vi "plc ios.vi"(7 "Calibpath":path=path "D:/Data Break Padel Test Rig/config/Calib/Calib_Date.txt", 8 "error In":errorcluster, 11 "connection ID IN":refnum<k5>) -> (0 "error out":errorcluster, 3 "connection ID OUT":refnum<k5>)   [LabVIEW 2015]
uses:
  Calibration/calibration.ctl
panel:
  out "PLC INPUT":T1
  out "PLC OUTPUT":T2
  out "Data":u32[](array[numeric])
  in  "Stop Button":bool
  # "PLC I/O's Detail"
  # "X40\tSATRT PB\nX41\tEMERGENYY PB\nX42\tRESET PB\nX43\tHOME PB\nX44\tCONTROL ON SIGNAL\nX45\tAIR PRESSURE SIGNAL\nX46\tSAFETY SENSOR SIGNAL-1\nX47\tSAFETY SENSOR SIGNAL-2\nX48\tPART PRESENMT SENSOR\nX49\tCLAMP CYL-1 UP RS\nX4A\tCLAMP CYL-1 DWN RS\nX4B\tCLAMP CYL-2 UP RS\nX4C\tCLAMP CYL-2 DWN RS\nX4D\tSPRING HOLD CYL FWD RS\nX4E\tSPRING HOLD CYL REV RS\nX4F\tSLIDE CYL UP RS\nX50\tSLIDE CYL DWN RS\nX51\tFRONT SIMULATOR REV RS\nX52\tBACK SIMULATOR REV RS\nX53\tSERVO HOMING SENSOR\nX54\tSERVO FWD OVER TRAVEL\nX55\tSERVO REV OVER TRAVEL\nX56\tSERVO FAULT SIGNAL\nX57\tPANEL DOOR OPEN SIGNAL\nX58\tSPARE\nX59\tSPARE\nX5A\tSPARE\nX5B\tSPARE\nX5C\tSPARE\nX5D\tSPARE\nX5E\tSPARE\nX5F\tSPARE"
  # "ATMA AUTOTECH ENGINEERS PVT. LTD."
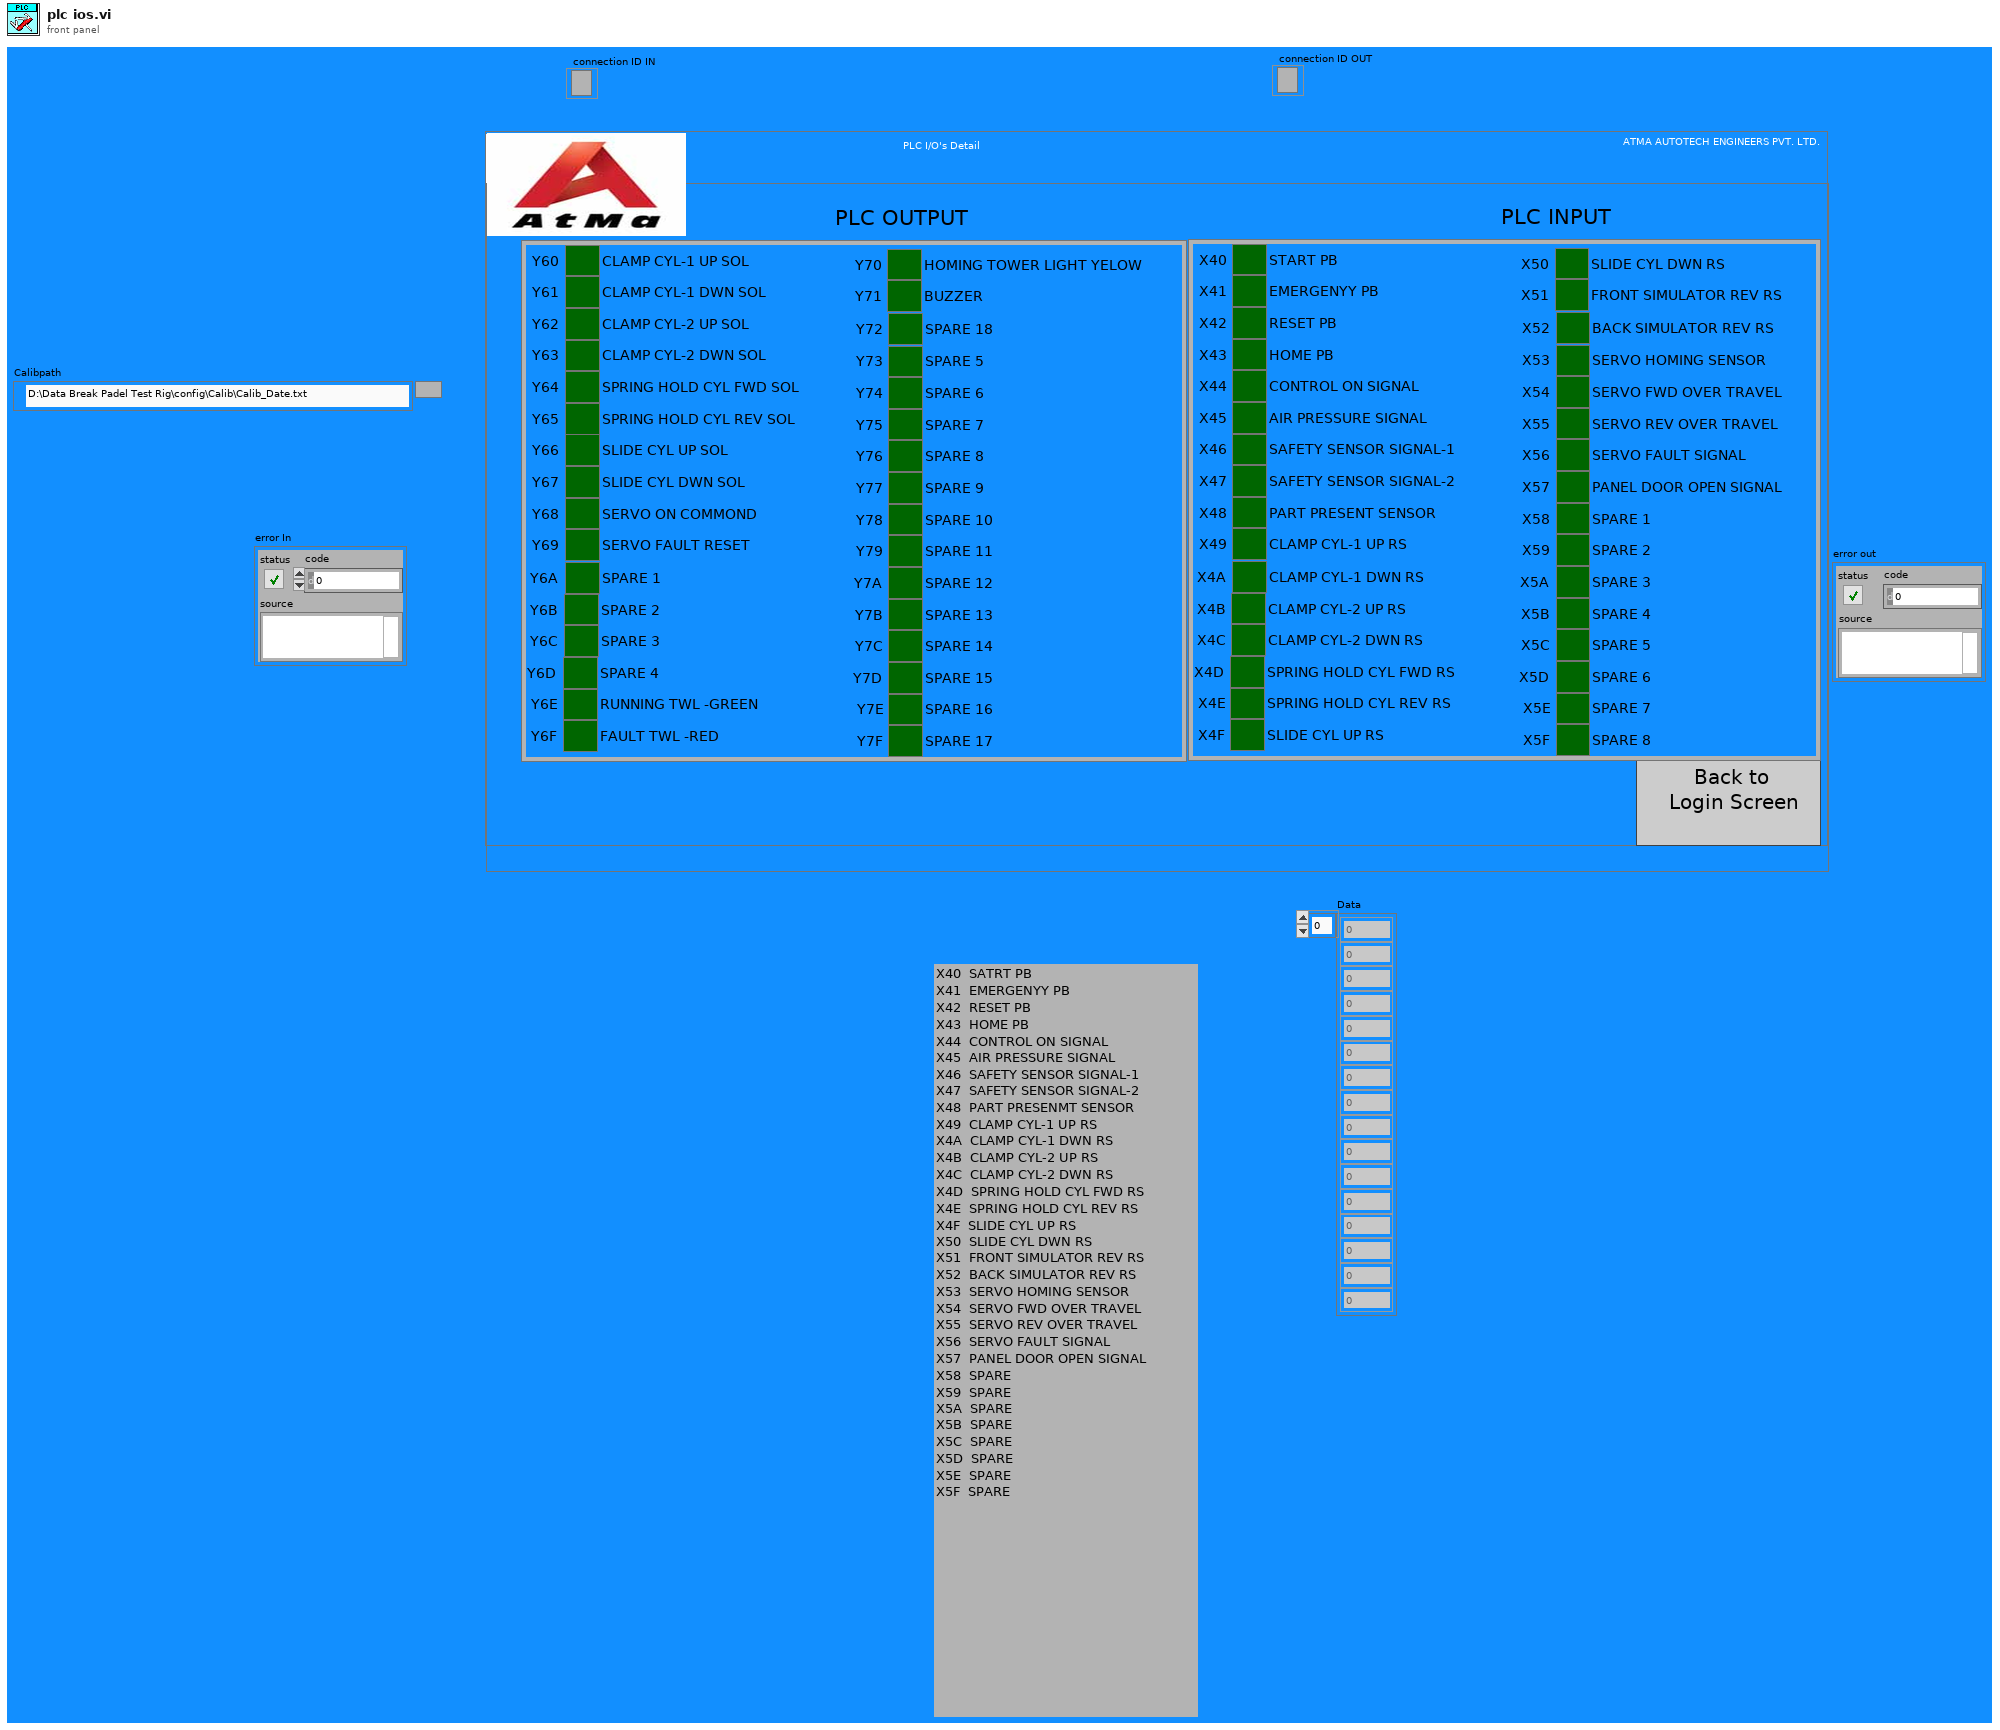
[diagram p1: front panel]
types:
  T1 = cluster{"START PB":bool, "EMERGENYY PB":bool, "RESET PB":bool, "HOME PB":bool, "CONTROL ON SIGNAL":bool, "AIR PRESSURE SIGNAL":bool, "SAFETY SENSOR SIGNAL-1":bool, "SAFETY SENSOR SIGNAL-2":bool, "PART PRESENT SENSOR":bool, "CLAMP CYL-1 UP RS":bool, "CLAMP CYL-1 DWN RS":bool, "CLAMP CYL-2 UP RS":bool, "CLAMP CYL-2 DWN RS":bool, "SPRING HOLD CYL FWD RS":bool, "SPRING HOLD CYL REV RS":bool, "SLIDE CYL UP RS":bool, "SLIDE CYL DWN RS":bool, "FRONT SIMULATOR REV RS":bool, "BACK SIMULATOR REV RS":bool, "SERVO HOMING SENSOR":bool, "SERVO FWD OVER TRAVEL":bool, "SERVO REV OVER TRAVEL":bool, "SERVO FAULT SIGNAL":bool, "PANEL DOOR OPEN SIGNAL":bool, "SPARE 1":bool, "SPARE 2":bool, "SPARE 3":bool, "SPARE 4":bool, "SPARE 5":bool, "SPARE 6":bool, "SPARE 7":bool, "SPARE 8":bool}
  T2 = cluster{"CLAMP CYL-1 UP SOL":bool, "CLAMP CYL-1 DWN SOL":bool, "CLAMP CYL-2 UP SOL":bool, "CLAMP CYL-2 DWN SOL":bool, "SPRING HOLD CYL FWD SOL":bool, "SPRING HOLD CYL REV SOL":bool, "SLIDE CYL UP SOL":bool, "SLIDE CYL DWN SOL":bool, "SERVO ON COMMOND":bool, "SERVO FAULT RESET":bool, "SPARE 1":bool, "SPARE 2":bool, "SPARE 3":bool, "SPARE 4":bool, "RUNNING TWL -GREEN":bool, "FAULT TWL -RED":bool, "HOMING TOWER LIGHT YELOW ":bool, "BUZZER":bool, "SPARE 18":bool, "SPARE 5":bool, "SPARE 6":bool, "SPARE 7":bool, "SPARE 8":bool, "SPARE 9":bool, "SPARE 10":bool, "SPARE 11":bool, "SPARE 12":bool, "SPARE 13":bool, "SPARE 14":bool, "SPARE 15":bool, "SPARE 16":bool, "SPARE 17":bool}
  T3 = typedef "calibration.ctl" = cluster{"Pressing Load":cluster{"Rating":dbl, "Multiplier":dbl, "Offset":dbl}, "Front Break Load":cluster{"Rating":dbl, "Multiplier":dbl, "Offset":dbl}, "Rear Break Load":cluster{"Rating":dbl, "Multiplier":dbl, "Offset":dbl}, "Front Break LVDT":cluster{"Rating":dbl, "Multiplier":dbl, "Offset":dbl}, "Rear Break LVDT":cluster{"Rating":dbl, "Multiplier":dbl, "Offset":dbl}, "AI 5":cluster{"Rating":dbl, "Multiplier":dbl, "Offset":dbl}, "AI 6":cluster{"Rating":dbl, "Multiplier":dbl, "Offset":dbl}, "AI 7":cluster{"Rating":dbl, "Multiplier":dbl, "Offset":dbl}}
  T4 = enum16{"open", "replace", "create", "open or create", "replace or create", "replace or create with confirmation"}
  T5 = cluster{"Rating":dbl, "Multiplier":dbl, "Offset":dbl}
  T6 = cluster{"DI 0-31[0]":bool, "DI 0-31[1]":bool, "DI 0-31[2]":bool, "DI 0-31[3]":bool, "DI 0-31[4]":bool, "DI 0-31[5]":bool, "DI 0-31[6]":bool, "DI 0-31[7]":bool, "DI 0-31[8]":bool, "DI 0-31[9]":bool, "DI 0-31[10]":bool, "DI 0-31[11]":bool, "DI 0-31[12]":bool, "DI 0-31[13]":bool, "DI 0-31[14]":bool, "DI 0-31[15]":bool, "DI 0-31[16]":bool, "DI 0-31[17]":bool, "DI 0-31[18]":bool, "DI 0-31[19]":bool, "DI 0-31[20]":bool, "DI 0-31[21]":bool, "DI 0-31[22]":bool, "DI 0-31[23]":bool, "DI 0-31[24]":bool, "DI 0-31[25]":bool, "DI 0-31[26]":bool, "DI 0-31[27]":bool, "DI 0-31[28]":bool, "DI 0-31[29]":bool, "DI 0-31[30]":bool, "DI 0-31[31]":bool}
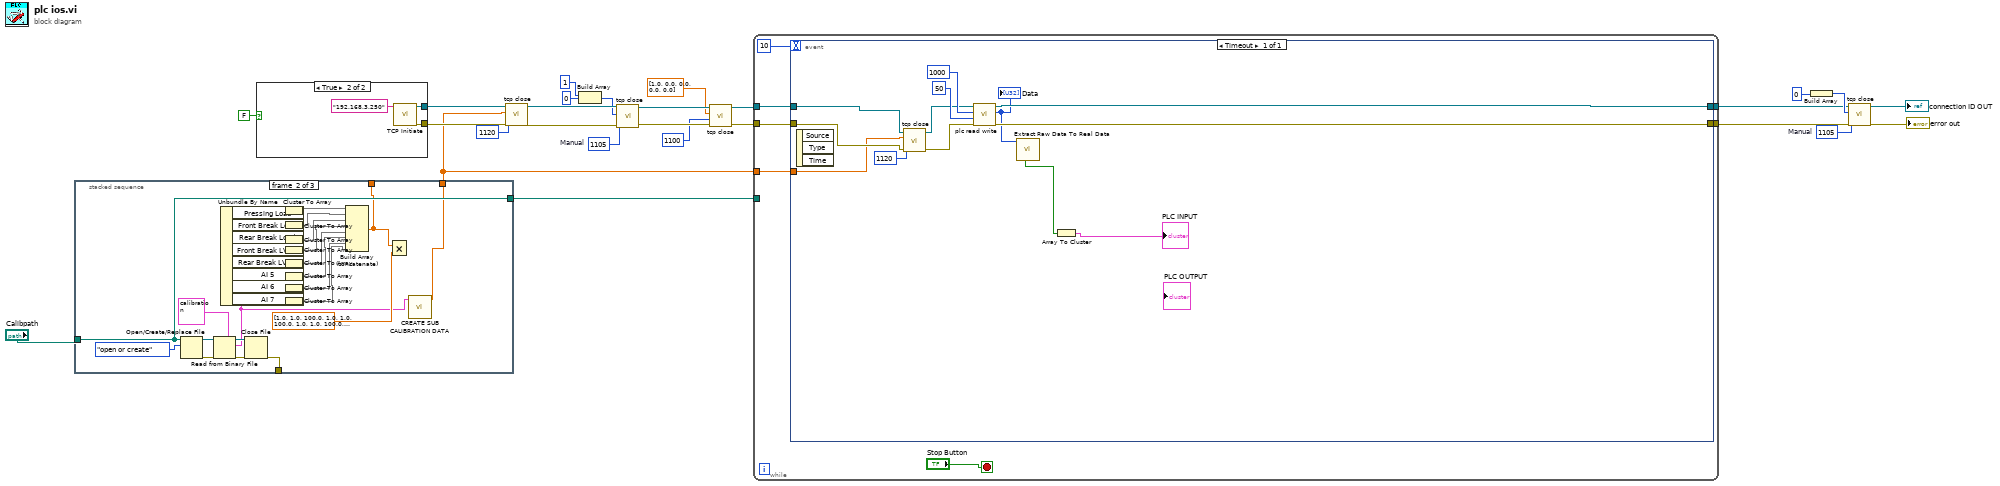
[diagram p0: block diagram]
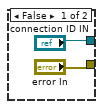
[diagram p2: hidden frame]
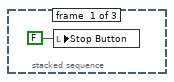
[diagram p3: hidden frame]
diagram:
  w11 = 1105  # Manual
  w19 = 1105  # Manual
  n1 = stacked-sequence {
    tunnel: "Calibpath" -> [_ w48 _]
    tunnel: [_ w48 _] -> w24
    tunnel: [_ w47 _] -> _
    tunnel: [_ w30 _] -> _
    tunnel: [_ w27 _] -> w6
    frame #0 {
      n2 = local write "Stop Button"(FALSE ("Stop Button")) -> ()
    }
    frame #1 {
      n3 = Open/Create/Replace File(file path (use dialog)=w48, operation (0:open)=T4."open or create") -> (refnum out=w52:refnum<file>, error out=w50:errorcluster)  [unwired: 4 in, 1 out]
      n4 = Read from Binary File(5:T3 {"Pressing Load"={"Rating"=0.0, "Multiplier"=0.0, "Offset"=0.0}, "Front Break Load"={"Rating"=0.0, "Multiplier"=0.0, "Offset"=0.0}, "Rear Break Load"={"Rating"=0.0, "Multiplier"=0.0, "Offset"=0.0}, "Front Break LVDT"={"Rating"=0.0, "Multiplier"=0.0, "Offset"=0.0}, "Rear Break LVDT"={"Rating"=0.0, "Multiplier"=0.0, "Offset"=0.0}, "AI 5"={"Rating"=0.0, "Multiplier"=0.0, "Offset"=0.0}, "AI 6"={"Rating"=0.0, "Multiplier"=0.0, "Offset"=0.0}, "AI 7"={"Rating"=0.0, "Multiplier"=0.0, "Offset"=0.0}} ("output cluster"), 8:w50, 11:w52) -> (0:w51:errorcluster, 2:w28:T3, 3:w53:refnum<file>)  [unwired: 3 in, 1 out]
      n5 = Unbundle By Name(w28) -> ("Pressing Load"=w46:T5, "Front Break Load"=w45:T5, "Rear Break Load"=w44:T5, "Front Break LVDT"=w43:T5, "Rear Break LVDT"=w39:T5, "AI 5"=w40:T5, "AI 6"=w41:T5, "AI 7"=w42:T5)
      n6 = Close File(refnum=w53, error in=w51) -> (error out=w47:errorcluster)  [unwired: 1 out]
      n7 = Cluster To Array(cluster=w46) -> (array=w38:dbl[])
      n8 = Cluster To Array(cluster=w45) -> (array=w37:dbl[])
      n9 = Cluster To Array(cluster=w44) -> (array=w36:dbl[])
      n10 = Cluster To Array(cluster=w43) -> (array=w35:dbl[])
      n11 = Cluster To Array(cluster=w39) -> (array=w34:dbl[])
      n12 = Cluster To Array(cluster=w40) -> (array=w33:dbl[])
      n13 = Cluster To Array(cluster=w41) -> (array=w32:dbl[])
      n14 = Cluster To Array(cluster=w42) -> (array=w31:dbl[])
      n15 = Build Array (concatenate)(w38, w37, w36, w35, w34, w33, w32, w31) -> (w30:dbl[])
      n16 = Multiply(x=w30, y=dbl[] [1.0, 1.0, 100.0, 1.0, 1.0, 100.0, 1.0, 1.0, 100.0, 1.0, 1.0, 100.0, 1.0, 1.0, 100.0, 1.0, 1.0, 100.0, 1.0, 1.0, 100.0, 1.0, 1.0, 100.0] ("initialized array")) -> ()  [unwired: 1 out]
      n17 = call "CREATE SUB CALIBRATION DATA.vi"("Calibration Factor"=w28) -> ("OUT"=w27:dbl[])  [unwired: 10 in]
    }
    frame #2 {
    }
  }
  n18 = case shown="True" FALSE {
    tunnel: ["connection ID IN" w59] -> w21
    tunnel: ["error In" w58] -> w20
    frame False {
    }
    frame True {
      n19 = call "TCP Initiate.vi"("IP ADDRESS"="192.168.3.250") -> ("error out"=w58:errorcluster, "connection ID"=w59:refnum<k5>)  [unwired: 9 in]
    }
  }
  n20 = call "tcp close.vi"("error in"=w20, "Address"=1120, "Write Data"=w6, "connection ID IN"=w21) -> ("error out"=w18:errorcluster, "connection ID out"=w17:refnum<k5>)  [unwired: 6 in]
  n21 = Build Array(1 ("length"), 0 ("element")) -> (w15:i32[])
  n22 = call "tcp close.vi"("error in"=w18, "Address"=w19, "Write Data"=w15, "connection ID IN"=w17) -> ("error out"=w16:errorcluster, "connection ID out"=w4:refnum<k5>)  [unwired: 6 in]
  n23 = call "tcp close.vi"("Address"=1100, "Write Data"=sgl[] [1.0, 0.0, 0.0, 0.0, 0.0] ("Write Data 2"), "connection ID IN"=w4) -> ("connection ID out"=w3:refnum<k5>)  [unwired: 7 in, 1 out]
  n24 = while {
    tunnel: w24 -> [_]
    tunnel: w3 -> [w65]
    tunnel: w16 -> [w64]
    tunnel: [w63] -> w10
    tunnel: [w62] -> w9
    tunnel: w6 -> [w60]
    stop <- "Stop Button" stop-if-true
    n25 = event shown="[0] Timeout" {
      selector: _ -> [_]
      dyn-events: _ -> [_]
      timeout: 10 -> [_]
      tunnel: w65 -> [w73]
      tunnel: w64 -> [w71]
      tunnel: [w77] -> w63
      tunnel: [w76] -> w62
      tunnel: w60 -> [w69]
      event Timeout {
        n26 = event-data() -> ()  [unwired: 1 in, 3 out]
        n27 = call "tcp close.vi"("error in"=w71, "Address"=1120, "Write Data"=w69, "connection ID IN"=w73) -> ("error out"=w70:errorcluster, "connection ID out"=w72:refnum<k5>)  [unwired: 6 in]
        n28 = call "plc read write.vi"("error In"=w70, "Length"=50, "Start Address"=1000, "connection ID IN"=w72) -> ("error out"=w76:errorcluster, "Data"=w75:u32[], "connection ID OUT"=w77:refnum<k5>)  [unwired: 5 in]
        "Data" <- w75
        n29 = call "Extract Raw Data To Real Data.vi"("data"=w75) -> ("DI 0-31"=w68:bool[])  [unwired: 3 in, 7 out]
        n30 = Array To Cluster(array=w68) -> (cluster=→"PLC INPUT":T6)
      }
    }
  }
  n31 = Build Array(0 ("length")) -> (w12:i32[])
  n32 = call "tcp close.vi"("error in"=w9, "Address"=w11, "Write Data"=w12, "connection ID IN"=w10) -> ("error out"=→"error out":errorcluster, "connection ID out"=→"connection ID OUT":refnum<k5>)  [unwired: 6 in]
